vi "Climb Controller.vi"(8 "error in":errorcluster) -> ()   [LabVIEW 2019]
doc: "This VI executes continuously carrying out the current operation and responding to updates or new operations. It will often contain the timing or control code that is difficult to place directly in TeleOp. This VI generally opens all sensors and motors and isolates the rest of the robot code from knowing how the operations are carried out."
uses:
  <vilib>/Rock Robotics/WPI/Framework/Completion Status.ctl
  Climb Setpoints.ctl
  Climb Operations.ctl
  <vilib>/Rock Robotics/WPI/ThirdParty/REV Robotics/SPARK MAX/Typedef/Spark MAX Motor Type.ctl
  <vilib>/Rock Robotics/WPI/ThirdParty/REV Robotics/SPARK MAX/Typedef/Spark MAX Idle Mode.ctl
  <vilib>/Rock Robotics/WPI/ThirdParty/REV Robotics/SPARK MAX/Typedef/Spark MAX Control Type.ctl
  Climb Published Globals.vi
panel:
  out "Setpoints":T1(graph)
  in  "Motor CAN IDs":cluster{"Lift":u8, "Spool":u8}={"Lift"=15, "Spool"=4}
  in  "Interactive Values":T2
  out "Current\nCmd":string
  in  "Buttons":cluster{"Execute Cmd":bool, "Abort Cmd":bool}
  out "Command Timing":cluster{"Start Time (ms)":u32, "Iterations":i32}
  out "Status":T4
  # "Tip: It may be helpful to observe inputs and sensor values.\nYou may also want to display tuning or debugging controls."
  # "Interactive Command: You may fill in the settings for a command\nand schedule it with the Execute button. You can observe and abort\nany command while fine tuning the code for the controller."
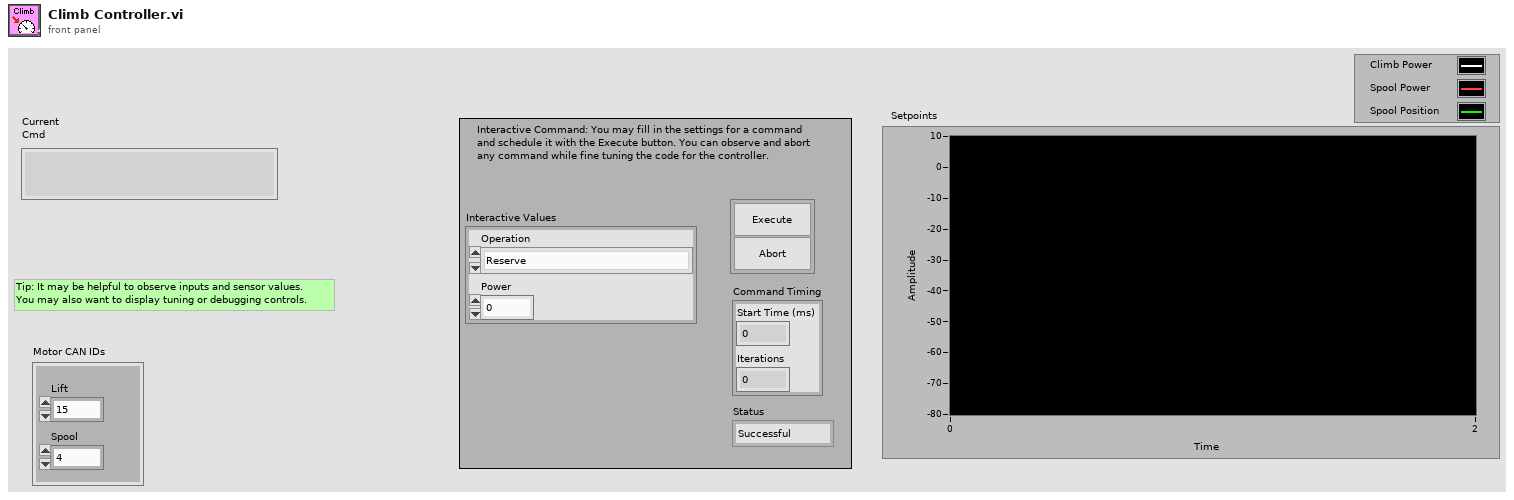
[diagram p1: front panel]
types:
  T1 = cluster{"Climb Power":dbl, "Spool Power":dbl, "Spool Power 2":dbl}
  T2 = typedef "Climb Setpoints.ctl" = cluster{"Operation":T3, "Power":dbl}
  T3 = typedef "Climb Operations.ctl" = enum16{"Reserve", "Read Current", "Immediate", "Climb Immediate", "Spool Immediate"}
  T4 = typedef "Completion Status.ctl" = enum16{"Successful", "Aborted", "Incomplete"}
  T5 = typedef "Spark MAX Idle Mode.ctl" = enum16{"Coast", "Brake"}
  T6 = typedef "Spark MAX Motor Type.ctl" = enum16{"Brushed", "Brushless"}
  T7 = typedef "WPI_MotorControlDeviceRef.ctl" = cluster{"DeviceStatus":errorcluster, "Type":T8, "PWM":cluster{"PWM Channel":T9, "DeadBand":T10}, "CAN":cluster{"Device Number":u8, "SetOutput VI Ref":variant, "GetOutput VI Ref":variant, "Enable VI Ref":variant, "Disable VI Ref":variant, "Data":variant}, "Invert":bool, "DIO PWM":cluster{"PWM \"Enable\" Channel":T9, "DIOChannel":T11, "PWM Rate":dbl}}
  T8 = typedef "WPI_MotorControlType.ctl" = enum16{"PWM", "CAN", "DIO PWM"}
  T9 = typedef "FPGA_DIOPWMChannel.ctl" = enum8{"PWM 0", "PWM 1", "PWM 2", "PWM 3", "PWM 4", "PWM 5", "PWM 6", "PWM 7", "PWM 8", "PWM 9", "PWM MXP 0", "PWM MXP 1", "PWM MXP 2", "PWM MXP 3", "PWM MXP 4", "PWM MXP 5", "PWM MXP 6", "PWM MXP 7", "PWM MXP 8", "PWM MXP 9", "Invalid"}
  T10 = typedef "WPI_PWMDeadband.ctl" = cluster{"Name":string, "maxPositivePwm":i32, "minPositivePwm":i32, "centerPwm":i32, "maxNegativePwm":i32, "minNegativePwm":i32, "angularRange":u16}
  T11 = typedef "FPGA_DIOChannel.ctl" = enum8{"DIO 0", "DIO 1", "DIO 2", "DIO 3", "DIO 4", "DIO 5", "DIO 6", "DIO 7", "DIO 8", "DIO 9", "DIO MXP 0", "DIO MXP 1", "DIO MXP 2", "DIO MXP 3", "DIO MXP 4", "DIO MXP 5", "DIO MXP 6", "DIO MXP 7", "DIO MXP 8", "DIO MXP 9", "DIO MXP 10", "DIO MXP 11", "DIO MXP 12", "DIO MXP 13", "DIO MXP 14", "DIO MXP 15", "SPI Port CS1", "SPI Port CS2", "SPI Port CS3", "SPI Port MISO", "SPI Port MOSI", "Invalid"}
  T12 = typedef "Command Status Info.ctl" = cluster{"Name":string, "Status":T4, "notifier out":T13}
  T13 = typedef "Completion Notifier.ctl" = refnum<notifier>
  T14 = cluster{"Current Command":T2, "Command Timing":cluster{"Start Time (ms)":u32, "Iterations":i32}, "Command Arguments":cluster{"Command Info":T12, "Description":string, "Default Command":T2, "queue out":refnum<queue>, "Subsystem Name":string}}
  T15 = cluster{"Climb Power":dbl, "Spool Power":dbl, "Spool Position":dbl}
  T16 = typedef "Spark MAX Control Type.ctl" = enum16{"Percent VBus", "Voltage", "Velocity", "Position", "Smart Motion", "Current", "Smart Velocity"}
  T17 = cluster{"P Gain":dbl, "I Gain":dbl, "D Gain":dbl, "F Gain":dbl, "I Zone":dbl, "Min Output":dbl, "Max Output":dbl}
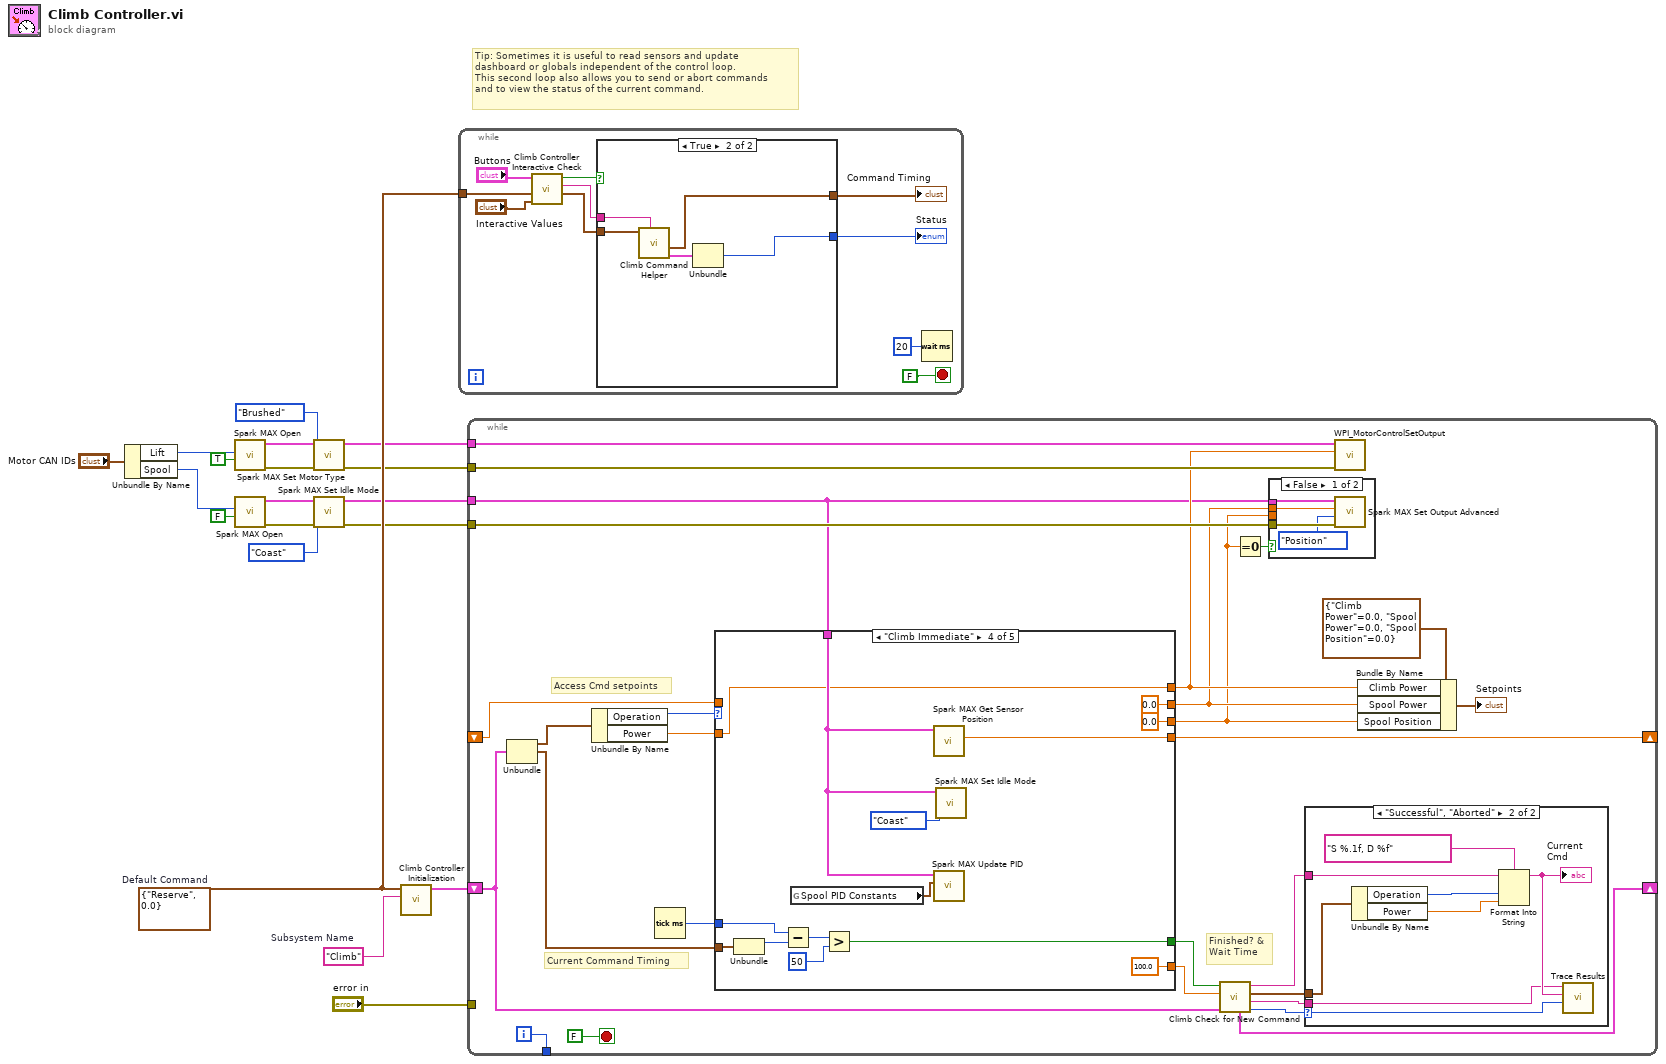
[diagram p0: block diagram]
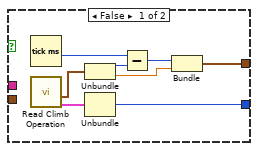
[diagram p2: hidden frame]
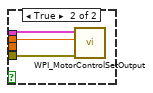
[diagram p3: hidden frame]
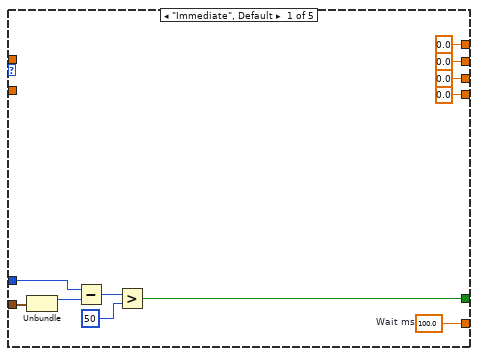
[diagram p5: hidden frame]
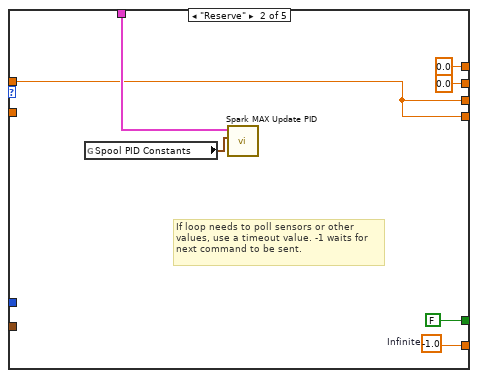
[diagram p6: hidden frame]
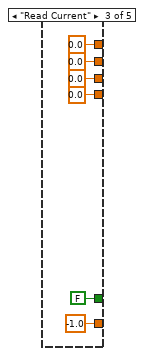
[diagram p7: hidden frame]
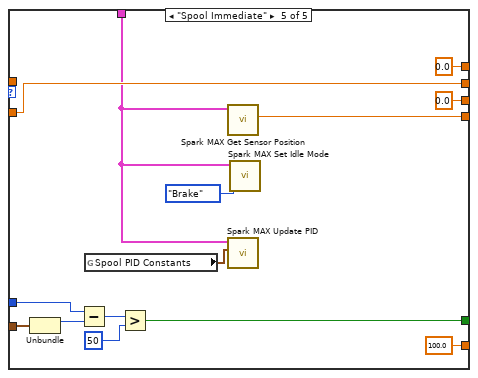
[diagram p8: hidden frame]
diagram:
  w16 = T2 {"Operation"=enum."Reserve", "Power"=0.0}  # Default Command
  w17 = "Climb"  # Subsystem Name
  # "Tip: Sometimes it is useful to read sensors and update\ndashboard or globals independent of the control loop.\nThis second loop also allows you to send or abort commands\nand to view the status of the current command."
  n1 = Unbundle By Name("Motor CAN IDs") -> ("Lift"=w14:u8, "Spool"=w13:u8)
  n2 = call <vilib>:"Spark MAX Open.vi"("Invert"=TRUE, "Device Number"=w14) -> ("error out"=w9:errorcluster, "MotorControlDeviceRef"=w10:T7)  [unwired: 8 in]
  n3 = call <vilib>:"Spark MAX Open.vi"("Invert"=FALSE, "Device Number"=w13) -> ("error out"=w4:errorcluster, "MotorControlDeviceRef"=w5:T7)  [unwired: 8 in]
  n4 = call <vilib>:"Spark MAX Set Motor Type.vi"("error in (no error)"=w9, "Motor Type"=Spark_MAX_Motor_Type."Brushed", "MotorControlDevRef"=w10) -> ("error out"=w7:errorcluster, "MotorControlDeviceRef"=w8:T7)  [unwired: 7 in]
  n5 = call <vilib>:"Spark MAX Set Idle Mode.vi"("error in (no error)"=w4, "Idle Mode"=Spark_MAX_Idle_Mode."Coast", "MotorControlDeviceRef in"=w5) -> ("error out"=w2:errorcluster, "MotorControlDeviceRef out"=w3:T7)  [unwired: 7 in]
  n6 = call "Climb Controller Initialization.vi"("Subsystem Name"=w17, "Default Command"=w16) -> ("Current Command"=w18:T14)  [unwired: 9 in]
  n7 = while {
    tunnel: w16 -> [w26]
    stop <- FALSE stop-if-true
    n8 = call "Climb Controller Interactive Check.vi"("Interactive Command in"="Interactive Values", "Default Command"=w26, "Buttons"="Buttons") -> ("Interactive Command out"=w23:T2, "Trace String"=w24:string, "Schedule"=w25:bool)  [unwired: 6 in]
    n9 = case shown="True" w25 {
      tunnel: [w37 w42] -> w22
      tunnel: w23 -> [_ w40]
      tunnel: [w33 w38] -> w21
      tunnel: w24 -> [_ w41]
      frame False {
        n10 = Tick Count (ms)() -> (millisecond timer value=w32:u32)
        n11 = call "Read Climb Operation.vi"() -> ("Command Info"=w30:T12, "SubSystem Data"=w31:T2)  [unwired: 9 in, 1 out]
        n12 = Unbundle(w31) -> ("Operation"=w36:T3, "Power"=w34:dbl)
        n13 = Unbundle(w30) -> ("Status"=w37:T4)  [unwired: 2 out]
        n14 = Subtract(x=w32, y=w36) -> (x-y=w35:u32)
        n15 = Bundle(w35, "Power"=w34) -> (w33:cluster{u32, "Power":dbl})  [unwired: 1 in]
      }
      frame True {
        n16 = call "Climb Command Helper.vi"("Description"=w41, "SubSystem Data"=w40) -> ("Command Info Out"=w39:T12, "Command Timing"=w38:cluster{"Start Time (ms)":u32, "Iterations":i32})  [unwired: 7 in, 1 out]
        n17 = Unbundle(w39) -> ("Status"=w42:T4)  [unwired: 2 out]
      }
    }
    "Status" <- w22
    "Command Timing" <- w21
    n18 = Wait (ms)(milliseconds to wait=u32 20) -> ()  [unwired: 1 out]
  }
  n19 = while {
    shift-right: [w62] -> _
    shift-left: w18 -> [w55]
    tunnel: [w68] -> _
    tunnel: "error in" -> [_]
    tunnel: w3 -> [w47]
    tunnel: w2 -> [w54]
    tunnel: w8 -> [w53]
    tunnel: w7 -> [w52]
    shift-right: [w46] -> _
    shift-left: _ -> [w45]
    i -> [w68]
    stop <- FALSE stop-if-true
    # "Current Command Timing"
    # "Access Cmd setpoints"
    # "Finished? &\nWait Time"
    n20 = Unbundle(w55) -> ("Current Command"=w67:T2, "Command Timing"=w63:cluster{"Start Time (ms)":u32, "Iterations":i32})  [unwired: 1 out]
    n21 = Unbundle By Name(w67) -> ("Operation"=w66:T3, "Power"=w65:dbl)
    n22 = Tick Count (ms)() -> (millisecond timer value=w64:u32)
    n23 = case shown="\"Climb Immediate\"" w66 {
      tunnel: [w95 w102 -1.0 ("Infinite") 100.0 ("Infinite") 100.0 ("Infinite")] -> w60
      tunnel: [w89 FALSE ("ignore previous (F)") FALSE ("ignore previous (F)") w117 w131] -> w61
      tunnel: w63 -> [w91 _ _ w118 w132]
      tunnel: w65 -> [_ _ _ w109 w128]
      tunnel: w64 -> [w90 _ _ w119 w133]
      tunnel: [0.0 ("Output") 0.0 ("Output") 0.0 ("Output") w109 0.0 ("Output")] -> w49
      tunnel: [0.0 ("Power") 0.0 ("Power") 0.0 ("Power") 0.0 ("Output") w128] -> w48
      tunnel: [0.0 ("Sensor Position") w96 0.0 ("Sensor Position") 0.0 ("Sensor Position") 0.0 ("Sensor Position")] -> w44
      tunnel: w47 -> [_ w99 _ w110 w123]
      tunnel: [0.0 ("Sensor Position") w96 0.0 ("Sensor Position") w115 w130] -> w46
      tunnel: w45 -> [_ w96 _ _ _]
      frame "Immediate", Default {
        w95 = 100.0  # Wait ms
        n24 = Unbundle(w91) -> ("Start Time (ms)"=w94:u32)  [unwired: 1 out]
        n25 = Subtract(x=w90, y=w94) -> (x-y=w93:u32)
        n26 = Greater?(x=w93, y=u8 50 ("Left Motor")) -> (0:w89:bool)
      }
      frame "Reserve" {
        w102 = -1.0  # Infinite
        # "If loop needs to poll sensors or other\nvalues, use a timeout value. -1 waits for\nnext command to be sent."
        n27 = global read "Climb Published Globals.vi" "Spool PID Constants"() -> (w100:T17)
        n28 = call "Spark MAX Update PID.vi"("MotorControlDeviceRef"=w99, "PID Constants"=w100) -> ()  [unwired: 8 in]
      }
      frame "Read Current" {
      }
      frame "Climb Immediate" {
        n29 = Unbundle(w118) -> ("Start Time (ms)"=w121:u32)  [unwired: 1 out]
        n30 = Subtract(x=w119, y=w121) -> (x-y=w122:u32)
        n31 = global read "Climb Published Globals.vi" "Spool PID Constants"() -> (w114:T17)
        n32 = Greater?(x=w122, y=u8 50 ("Left Motor")) -> (0:w117:bool)
        n33 = call <vilib>:"Spark MAX Get Sensor Position.vi"("MotorControlDevRef in"=w110) -> ("Sensor Position"=w115:dbl)  [unwired: 7 in, 3 out]
        n34 = call "Spark MAX Update PID.vi"("MotorControlDeviceRef"=w110, "PID Constants"=w114) -> ()  [unwired: 8 in]
        n35 = call <vilib>:"Spark MAX Set Idle Mode.vi"("Idle Mode"=Spark_MAX_Idle_Mode."Coast", "MotorControlDeviceRef in"=w110) -> ()  [unwired: 8 in, 2 out]
      }
      frame "Spool Immediate" {
        n36 = Unbundle(w132) -> ("Start Time (ms)"=w135:u32)  [unwired: 1 out]
        n37 = Subtract(x=w133, y=w135) -> (x-y=w136:u32)
        n38 = global read "Climb Published Globals.vi" "Spool PID Constants"() -> (w127:T17)
        n39 = Greater?(x=w136, y=u8 50 ("Left Motor")) -> (0:w131:bool)
        n40 = call <vilib>:"Spark MAX Get Sensor Position.vi"("MotorControlDevRef in"=w123) -> ("Sensor Position"=w130:dbl)  [unwired: 7 in, 3 out]
        n41 = call "Spark MAX Update PID.vi"("MotorControlDeviceRef"=w123, "PID Constants"=w127) -> ()  [unwired: 8 in]
        n42 = call <vilib>:"Spark MAX Set Idle Mode.vi"("Idle Mode"=Spark_MAX_Idle_Mode."Brake", "MotorControlDeviceRef in"=w123) -> ()  [unwired: 8 in, 2 out]
      }
    }
    n43 = call "Climb Check for New Command.vi"("Current Command"=w55, "Wait time (ms)"=w60, "Finished?"=w61) -> ("Completion"=w56:T4, "Subsystem Name"=w57:string, "Current Command"=w58:T2, "Initial Trace String"=w59:string, "NextCommand"=w62:T14)  [unwired: 4 in]
    n44 = Equal To 0?(x=w44) -> (x = 0?=w43:bool)
    n45 = case shown="False" w43 {
      tunnel: w47 -> [w72 w76]
      tunnel: w54 -> [w73 w75]
      tunnel: w48 -> [_ w74]
      tunnel: w44 -> [w70 _]
      frame False {
        n46 = call <vilib>:"Spark MAX Set Output Advanced.vi"("error in (no error)"=w73, "Control Mode"=Spark_MAX_Control_Type."Position", "Setpoint"=w70, "MotorControlDevRef"=w72) -> ()  [unwired: 6 in, 2 out]
      }
      frame True {
        n47 = call <vilib>:"WPI_MotorControlSetOutput.vi"("error in (no error)"=w75, "Output"=w74, "MotorControlDevRef"=w76) -> ()  [unwired: 6 in, 3 out]
      }
    }
    n48 = case shown="\"Successful\", \"Aborted\"" w56 {
      selector: w56 -> [_ w84]
      tunnel: w59 -> [_ w80]
      tunnel: w58 -> [_ w81]
      tunnel: w57 -> [_ w77]
      frame "Incomplete", Default {
        # "Continuing current command"
      }
      frame "Successful", "Aborted" {
        # "Report and setup for next command"
        n49 = Unbundle By Name(w81) -> ("Operation"=w83:T3, "Power"=w78:dbl)
        n50 = Format Into String(format string="S %.1f, D %f", initial string=w80, w83, w78) -> (resulting string=w79:string)  [unwired: 1 in, 1 out]
        "Current\nCmd" <- w79
        n51 = call <vilib>:"Trace Results.vi"("Status of previous command"=w84, "Description"=w79, "Subsystem"=w77) -> ()  [unwired: 9 in]
      }
    }
    n52 = call <vilib>:"WPI_MotorControlSetOutput.vi"("error in (no error)"=w52, "Output"=w49, "MotorControlDevRef"=w53) -> ()  [unwired: 6 in, 3 out]
    n53 = Bundle By Name(cluster=T15 {"Climb Power"=0.0, "Spool Power"=0.0, "Spool Position"=0.0} ("Setpoints"), "Climb Power"=w49, "Spool Power"=w48, "Spool Position"=w44) -> (→"Setpoints":T15)
  }
